vi "onReadPlatanoConfiguration.vi"(7 "Section (default)":string, 8 "error in (no error)":errorcluster, 10 "Config Map in":map{string, string}(c390), 11 "Platano in":refnum<class "Platano.lvclass">) -> (0 "error out":errorcluster, 2 "Config Map out":map{string, string}(c390), 3 "Platano out":refnum<class "Platano.lvclass">)   [LabVIEW 2021, in "Bananas.lvlib" / "Platano.lvclass"]
uses:
  Platano.lvclass
  <vilib>/Utility/sysdir.llb/System Directory Type.ctl
  <vilib>/Utility/config.llb/Read Key (String).vi
  <vilib>/Utility/config.llb/NI_LVConfig.lvlib
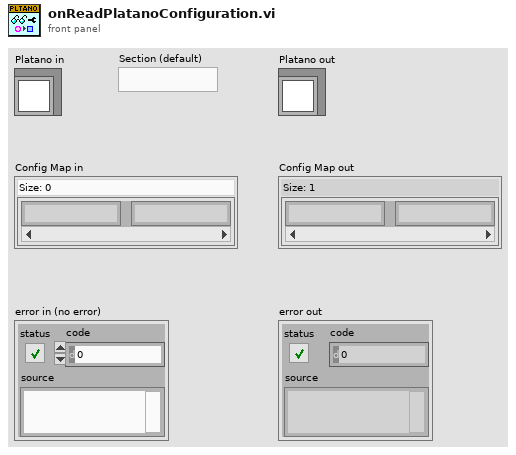
[diagram p1: front panel]
types:
  T1 = enum16{"open", "replace", "create", "open or create", "replace or create", "replace or create with confirmation"}
  T2 = typedef "System Directory Type.ctl" = i32
  T3 = typedef "NI_LVConfig.lvlib/Config Data RefNum.ctl" = refnum<k1>
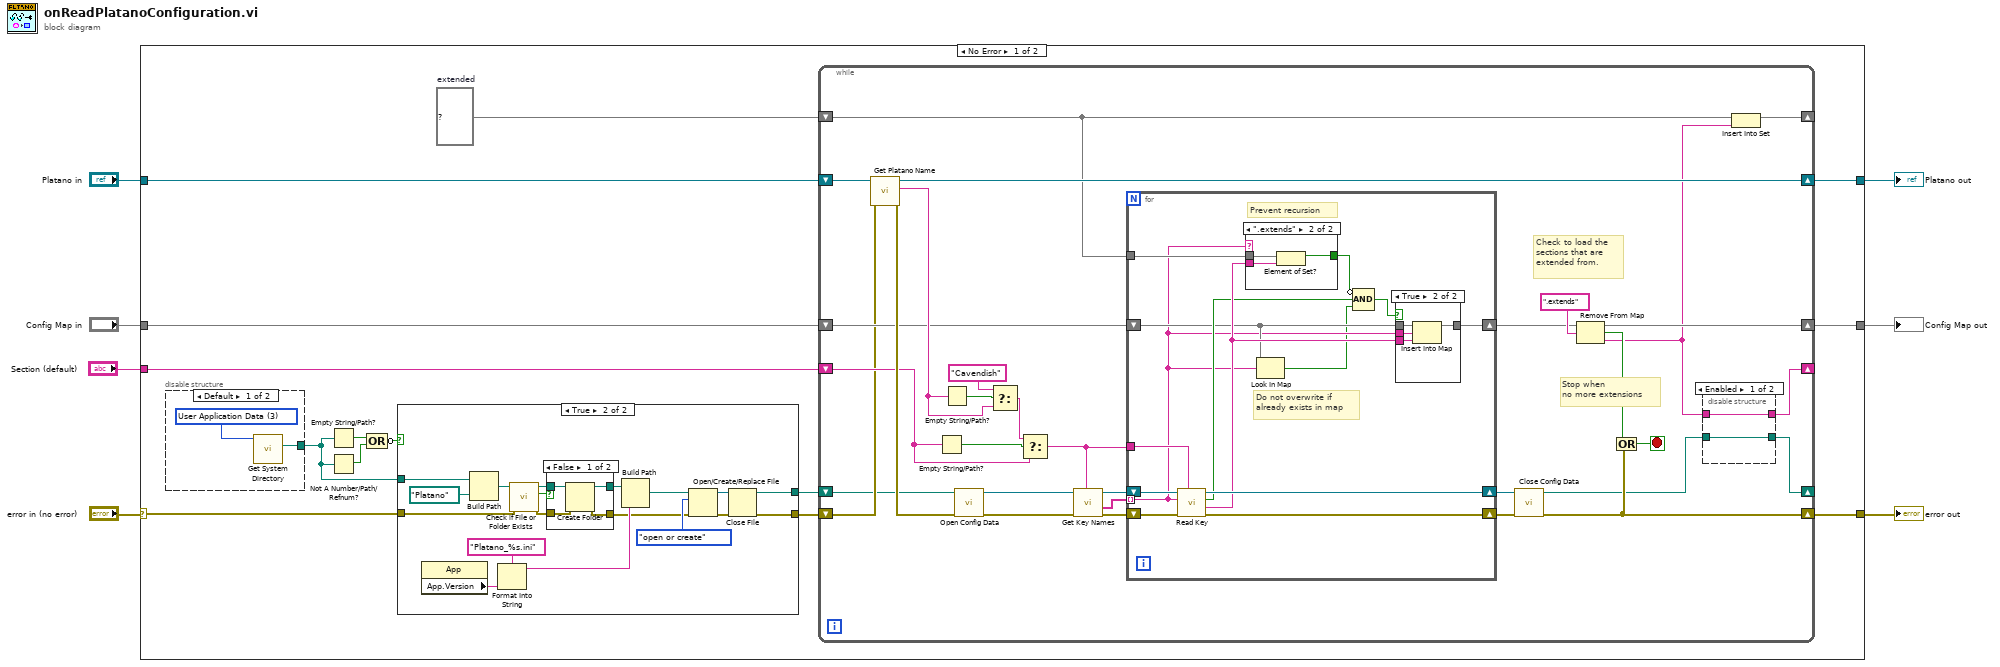
[diagram p0: block diagram]
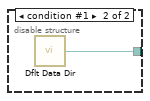
[diagram p2: hidden frame]
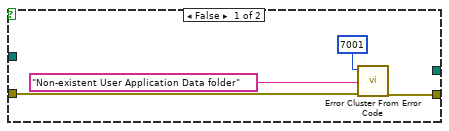
[diagram p3: hidden frame]
diagram:
  n1 = case shown="No Error" "error in (no error)" {
    selector: "error in (no error)" -> [w9 w111]
    tunnel: [w19 w111] -> w7
    tunnel: "Config Map in" -> [w18 w110]
    tunnel: [w17 w110] -> w4
    tunnel: [w21 w109] -> w3
    tunnel: "Platano in" -> [w20 w109]
    tunnel: "Section (default)" -> [w16 _]
    frame No Error {
      w15 = set{string} {}  # extended
      n2 = disable-structure shown="Default" {
        disable-tunnel: [w23 w24] -> w12
        frame condition #0 (active) {
          w22 = T2 3 items=["User Home"=0, "User Desktop"=1, "User Documents"=2, "User Application Data"=3, "User Preferences"=4, "User Temporary"=5, "Public Documents"=6, "Public Application Data"=7, "Public Preferences"=8, "Public Cache"=13, "System Core Libraries"=9, "System Installed Libraries"=10, "Application Files"=11, "Boot Volume Root"=12] ("system directory type")
          n3 = call <vilib>:"Get System Directory.vi"("system directory type"=w22) -> ("system directory"=w23:path)  [unwired: 10 in]
        }
        frame condition #1 {
          n4 = call <vilib>:"Dflt Data Dir.vi"() -> ("App:Default Data Directory"=w24:path)
        }
      }
      n5 = Empty String/Path?(string/path=w12) -> (empty?=w13:bool)
      n6 = Not A Number/Path/Refnum?(number/path/refnum=w12) -> (NaN/Path/Refnum?=w14:bool)
      n7 = Compound Arithmetic op=OR(w13, w14) -> (invert w8:bool)
      n8 = case shown="True" w8 {
        tunnel: w12 -> [_ w42]
        tunnel: [_ w40] -> w11
        tunnel: [w28 w36] -> w10
        tunnel: w9 -> [w25 w32]
        frame False {
          n9 = call <vilib>:"Error Cluster From Error Code.vi"("error in (no error)"=w25, "error message (\"\")"="Non-existent User Application Data folder" ("error message (\"\")"), "error code (0)"=7001) -> ("error out"=w28:errorcluster)  [unwired: 6 in]
        }
        frame True {
          n10 = property class="App"() -> ("App.Version"=w45:string)  [unwired: 2 in, 2 out]
          n11 = Build Path(base path=w42, name or relative path=path "Platano") -> (appended path=w34:path)
          n12 = Format Into String(format string="Platano_%s.ini", w45) -> (resulting string=w43:string)  [unwired: 2 in, 1 out]
          n13 = call <vilib>:"Check if File or Folder Exists.vi"("error in (no error)"=w32, "path"=w34) -> ("error out"=w31:errorcluster, "file or folder exists?"=w29:bool, "dup path"=w33:path)  [unwired: 7 in]
          n14 = case shown="False" w29 {
            tunnel: [w50 w52] -> w35
            tunnel: w33 -> [w49 w52]
            tunnel: w31 -> [w48 w51]
            tunnel: [w47 w51] -> w30
            frame False {
              n15 = Create Folder(path (use dialog)=w49, error in=w48) -> (created path=w50:path, error out=w47:errorcluster)  [unwired: 1 in, 1 out]
            }
            frame True {
            }
          }
          n16 = Build Path(base path=w35, name or relative path=w43) -> (appended path=w39:path)
          n17 = Open/Create/Replace File(file path (use dialog)=w39, error in=w30, operation (0:open)=T1."open or create") -> (refnum out=w41:refnum<file>, error out=w37:errorcluster)  [unwired: 3 in, 1 out]
          n18 = Close File(refnum=w41, error in=w37) -> (path=w40:path, error out=w36:errorcluster)
        }
      }
      n19 = while {
        shift-right: [w61] -> w19
        shift-left: w10 -> [w63]
        shift-right: [w67] -> w21
        shift-left: w20 -> [w84]
        shift-right: [w64] -> w17
        shift-left: w18 -> [w73]
        shift-right: [w55] -> _
        shift-left: w15 -> [w54]
        shift-right: [w58] -> _
        shift-left: w16 -> [w70]
        shift-right: [w56] -> _
        shift-left: w11 -> [w62]
        stop <- w59 stop-if-true
        # "Check to load the\nsections that are\nextended from."
        # "Stop when\nno more extensions"
        n20 = call "Get Platano Name.vi"("error in (no error)"=w63, "Platano in"=w84) -> ("error out"=w83:errorcluster, "Varietal"=w80:string, "Platano out"=w67:refnum<class "Platano.lvclass">)  [unwired: 7 in]
        n21 = Empty String/Path?(string/path=w70) -> (empty?=w72:bool)
        n22 = Empty String/Path?(string/path=w80) -> (empty?=w81:bool)
        n23 = call <vilib>:"Open Config Data.vi"("error in (no error)"=w83, "configuration file path"=w62) -> ("error out"=w82:errorcluster, "refnum"=w79:T3)  [unwired: 7 in, 1 out]
        n24 = Select(t="Cavendish" ("format string"), s=w81, f=w80) -> (s? t:f=w69:string)
        n25 = Select(t=w69, s=w72, f=w70) -> (s? t:f=w68:string)
        n26 = call <vilib>:"Get Key Names.vi"("section"=w68, "error in (no error)"=w82, "refnum"=w79) -> ("error out"=w78:errorcluster, "key names"=w74:string[], "refnum out"=w77:T3)  [unwired: 5 in, 1 out]
        n27 = for {
          tunnel: w68 -> [w96]
          tunnel: w74 -> [w88] mode=indexing
          shift-right: [w98] -> w76
          shift-left: w78 -> [w100]
          shift-right: [w97] -> w75
          shift-left: w77 -> [w99]
          shift-right: [w95] -> w65
          shift-left: w73 -> [w89]
          tunnel: w54 -> [w94]
          # "Do not overwrite if\nalready exists in map"
          # "Prevent recursion"
          n28 = call-poly <vilib>:"Read Key.vi"("section"=w96, "error in (no error)"=w100, "key"=w88, "refnum"=w99) -> ("error out"=w98:errorcluster, "value"=w93:string, "found?"=w91:bool, "refnum out"=w97:T3)  [unwired: 4 in]
          n29 = case shown="\".extends\"" w88 {
            tunnel: w94 -> [_ w103]
            tunnel: w93 -> [_ w102]
            tunnel: [_ w101] -> w92
            frame Default {
            }
            frame ".extends" {
              n30 = Element of Set?(10:w102, 11:w103) -> (3:w101:bool)
            }
          }
          n31 = Look In Map(map=w89, key=w88) -> (key not found?=w87:bool)  [unwired: 1 in, 1 out]
          n32 = Compound Arithmetic op=AND(invert w92, w91, w87) -> (w90:bool)
          n33 = case shown="True" w90 {
            tunnel: w89 -> [w104 w108]
            tunnel: [w104 w107] -> w95
            tunnel: w93 -> [_ w106]
            tunnel: w88 -> [_ w105]
            frame False {
            }
            frame True {
              n34 = Insert Into Map(map in=w108, key=w105, value=w106) -> (map out=w107:map{string, string})  [unwired: 2 out]
            }
          }
        }
        n35 = call <vilib>:"Close Config Data.vi"("error in (no error)"=w76, "refnum"=w75) -> ("error out"=w61:errorcluster, "file path"=w57:path)  [unwired: 8 in]
        n36 = Remove From Map(10:".extends" ("key"), 11:w65) -> (1:w53:string, 2:w60:bool, 3:w64:map{string, string})
        n37 = Or(x=w60, y=w61) -> (x .or. y?=w59:bool)
        n38 = disable-structure shown="Enabled" {
          disable-tunnel: [w86 _] -> w58
          disable-tunnel: w53 -> [w86 _]
          disable-tunnel: [w85 _] -> w56
          disable-tunnel: w57 -> [w85 _]
          frame Enabled {
          }
          frame Disabled {
          }
        }
        n39 = Insert Into Set(10:w53, 11:w54) -> (3:w55:set{string})  [unwired: 1 out]
      }
    }
    frame Error {
    }
  }
  "Platano out" <- w3
  "Config Map out" <- w4
  "error out" <- w7
